vi "StaticWriteMemBlock(TimeStamp).vi"(8 "error in (no error)":errorcluster caption="错误输入（无错误）", 10 "输入值":timestamp, 11 "标签":string) -> (0 "error out":errorcluster caption="错误输出")   [LabVIEW 2012]
uses:
  MemBlock/MemBlock(TimeStamp).vi
  MemBlockTag/MemBlockTagList(TimeStamps).vi
  MemBlock.lvlib
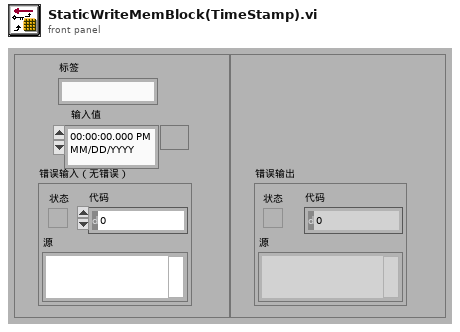
[diagram p1: front panel]
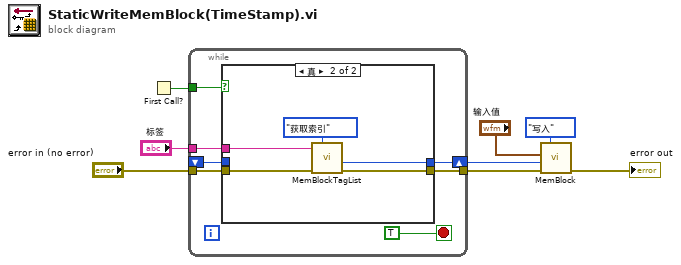
[diagram p0: block diagram]
diagram:
  n1 = First Call?() -> (First Call?: T/F=w2:bool)
  n2 = while {
    tunnel: [w15] -> w8
    tunnel: "error in (no error)" -> [w13]
    tunnel: w2 -> [w11]
    tunnel: "标签" -> [w10]
    shift-right: [w14] -> w7
    shift-left: _ -> [w9]
    stop <- TRUE stop-if-true
    n3 = case shown="真" w11 {
      tunnel: [w17 w21] -> w15
      tunnel: [w16 w20] -> w14
      tunnel: w13 -> [w17 w19]
      tunnel: w10 -> [_ w18]
      tunnel: w9 -> [w16 _]
      frame False {
      }
      frame True {
        n4 = call-poly "MemBlockTagList.vi"("方法"=enum16{"初始化", "获取索引"}."获取索引", "error in (no error)"=w19, "标签"=w18) -> ("error out"=w21:errorcluster, "标签索引"=w20:i32)  [unwired: 6 in, 1 out]
      }
    }
  }
  n5 = call-poly "MemBlock.vi"("方法"=enum16{"初始化", "读取", "读取全部", "写入"}."写入", "error in (no error)"=w8, "索引"=w7, "输入值"="输入值") -> ("error out"=→"error out":errorcluster)  [unwired: 5 in, 2 out]
